vi "Lakeshore_350_write.vi"(5 "File Reference":refnum<file>) -> ()   [LabVIEW 2019]
uses:
  Instrument_Setup.vi
  Global Variables/Data_Display_global.vi
panel:
  # "OFF"
  # "ON"
  # "OFF"
  # "ON"
  # "OFF"
  # "ON"
  # "OFF"
  # "ON"
  # "ON"
  # "OFF"
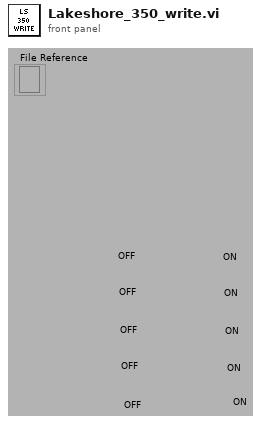
[diagram p1: front panel]
types:
  T1 = typedef "LS350-cluster.ctl" = cluster{"Setpoint":dbl, "Heater Output":dbl, "Setpoint control":dbl, "Enable Setpoint":bool, "LS350 T1":dbl, "LS350 T2":dbl, "LS350 T3":dbl, "LS350 T4":dbl, "LS350 R1":dbl, "LS350 R2":dbl, "LS350 R3":dbl, "LS350 R4":dbl}
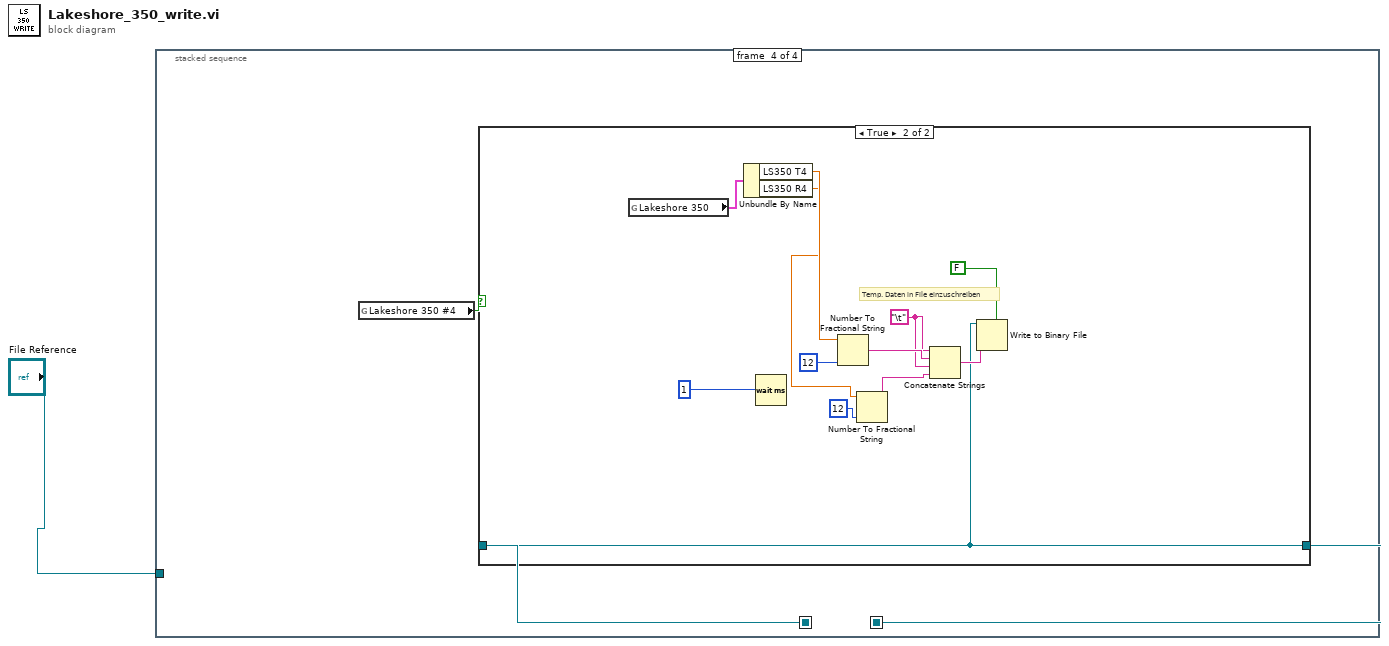
[diagram p0: block diagram]
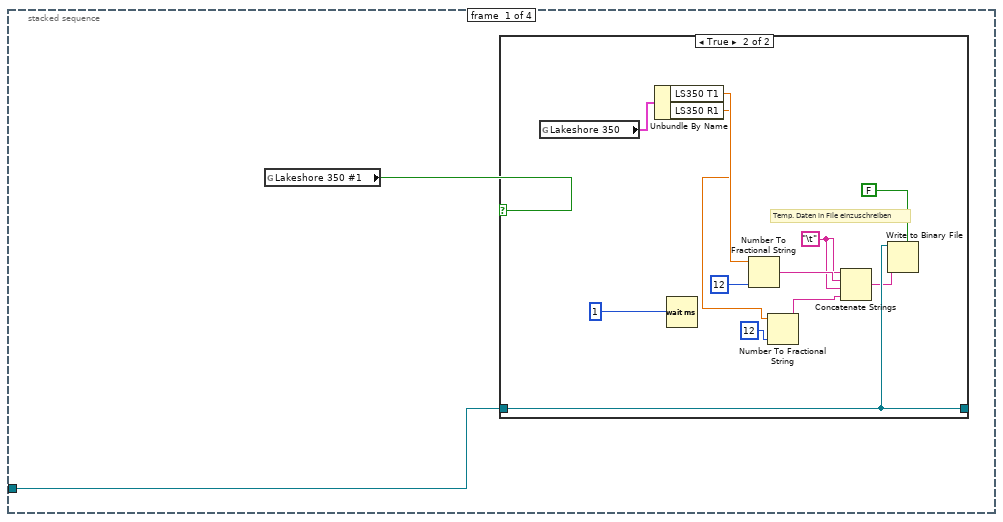
[diagram p2: hidden frame]
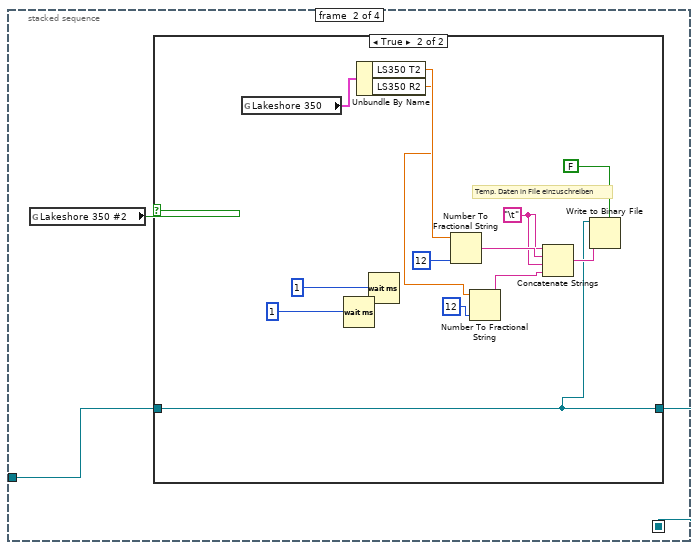
[diagram p4: hidden frame]
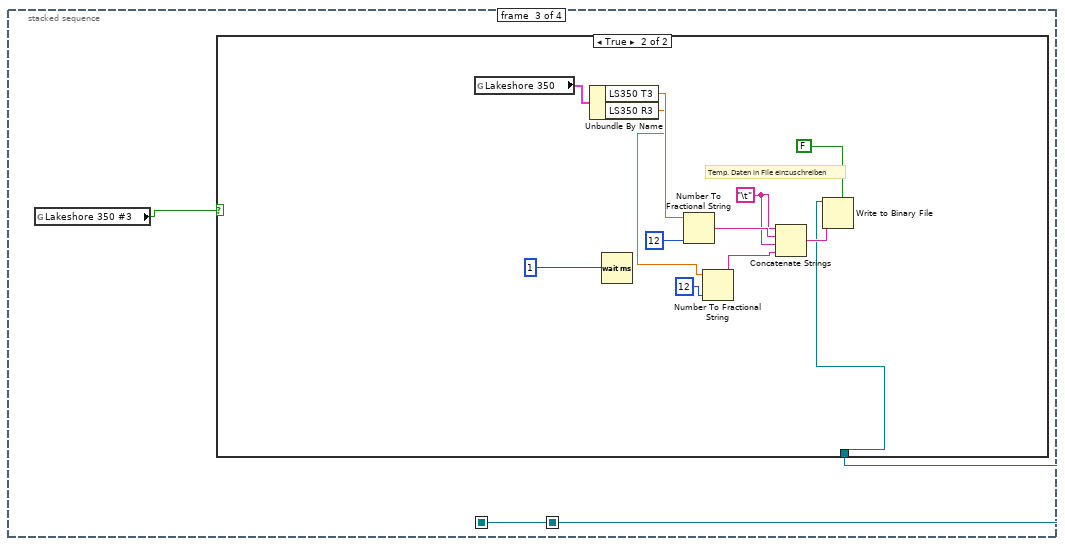
[diagram p6: hidden frame]
diagram:
  n1 = stacked-sequence {
    seq-local: [_ w18 _ _] -> [_ _ w34 w49]
    seq-local: [_ _ _ w48] -> [_ _ _ _]
    tunnel: "File Reference" -> [w2 w17 _ _]
    frame #0 {
      n2 = global read "Instrument_Setup.vi" "Lakeshore 350 #1"() -> (w3:bool)
      n3 = case shown="True" w3 {
        tunnel: w2 -> [w4 w16]
        tunnel: [w4 w16] -> _
        frame False {
        }
        frame True {
          w9 = "\t"
          # "Temp. Daten in File einzuschreiben"
          n4 = global read "Data_Display_global.vi" "Lakeshore 350"() -> (w7:T1)
          n5 = Unbundle By Name(w7) -> ("LS350 T1"=w6:dbl, "LS350 R1"=w5:dbl)
          n6 = Wait (ms)(milliseconds to wait=1) -> ()  [unwired: 1 out]
          n7 = Number To Fractional String(number=w6, precision (6)=i16 12) -> (F-format string=w13:string)  [unwired: 2 in]
          n8 = Number To Fractional String(number=w5, precision (6)=i16 12) -> (F-format string=w8:string)  [unwired: 2 in]
          n9 = Concatenate Strings(w9, w13, w9, w8) -> (w14:string)
          n10 = Write to Binary File ("Write File")(file (use dialog)=w16, data=w14, 5:FALSE ("prepend array or string size? (T)")) -> ()  [unwired: 3 in, 3 out]
        }
      }
    }
    frame #1 {
      n11 = global read "Instrument_Setup.vi" "Lakeshore 350 #2"() -> (w19:bool)
      n12 = case shown="True" w19 {
        tunnel: w17 -> [w20 w21]
        tunnel: [w20 w21] -> w18
        frame False {
        }
        frame True {
          w26 = "\t"
          # "Temp. Daten in File einzuschreiben"
          n13 = global read "Data_Display_global.vi" "Lakeshore 350"() -> (w24:T1)
          n14 = Wait (ms)(milliseconds to wait=1) -> ()  [unwired: 1 out]
          n15 = Unbundle By Name(w24) -> ("LS350 T2"=w23:dbl, "LS350 R2"=w22:dbl)
          n16 = Wait (ms)(milliseconds to wait=1) -> ()  [unwired: 1 out]
          n17 = Number To Fractional String(number=w23, precision (6)=i16 12) -> (F-format string=w30:string)  [unwired: 2 in]
          n18 = Number To Fractional String(number=w22, precision (6)=i16 12) -> (F-format string=w25:string)  [unwired: 2 in]
          n19 = Concatenate Strings(w26, w30, w26, w25) -> (w31:string)
          n20 = Write to Binary File ("Write File")(file (use dialog)=w21, data=w31, 5:FALSE ("prepend array or string size? (T)")) -> ()  [unwired: 3 in, 3 out]
        }
      }
    }
    frame #2 {
      n21 = global read "Instrument_Setup.vi" "Lakeshore 350 #3"() -> (w35:bool)
      n22 = case shown="True" w35 {
        tunnel: w34 -> [_ w36]
        frame False {
        }
        frame True {
          w41 = "\t"
          # "Temp. Daten in File einzuschreiben"
          n23 = global read "Data_Display_global.vi" "Lakeshore 350"() -> (w39:T1)
          n24 = Unbundle By Name(w39) -> ("LS350 T3"=w38:dbl, "LS350 R3"=w37:dbl)
          n25 = Wait (ms)(milliseconds to wait=1) -> ()  [unwired: 1 out]
          n26 = Number To Fractional String(number=w38, precision (6)=i16 12) -> (F-format string=w45:string)  [unwired: 2 in]
          n27 = Number To Fractional String(number=w37, precision (6)=i16 12) -> (F-format string=w40:string)  [unwired: 2 in]
          n28 = Concatenate Strings(w41, w45, w41, w40) -> (w46:string)
          n29 = Write to Binary File ("Write File")(file (use dialog)=w36, data=w46, 5:FALSE ("prepend array or string size? (T)")) -> ()  [unwired: 3 in, 3 out]
        }
      }
    }
    frame #3 {
      n30 = global read "Instrument_Setup.vi" "Lakeshore 350 #4"() -> (w50:bool)
      n31 = case shown="True" w50 {
        tunnel: w49 -> [w51 w52]
        tunnel: [w51 w52] -> w48
        frame False {
        }
        frame True {
          w57 = "\t"
          # "Temp. Daten in File einzuschreiben"
          n32 = global read "Data_Display_global.vi" "Lakeshore 350"() -> (w55:T1)
          n33 = Unbundle By Name(w55) -> ("LS350 T4"=w54:dbl, "LS350 R4"=w53:dbl)
          n34 = Wait (ms)(milliseconds to wait=1) -> ()  [unwired: 1 out]
          n35 = Number To Fractional String(number=w54, precision (6)=i16 12) -> (F-format string=w61:string)  [unwired: 2 in]
          n36 = Number To Fractional String(number=w53, precision (6)=i16 12) -> (F-format string=w56:string)  [unwired: 2 in]
          n37 = Concatenate Strings(w57, w61, w57, w56) -> (w62:string)
          n38 = Write to Binary File ("Write File")(file (use dialog)=w52, data=w62, 5:FALSE ("prepend array or string size? (T)")) -> ()  [unwired: 3 in, 3 out]
        }
      }
    }
  }
